vi "SubVI_EncTempl_003.vi"(0 "Encoder parameters":T1) -> (1 "Template images":picture[](array[picture]), 2 "Cluster templates":cluster{i32[], i32[][]})   [LabVIEW 2018]
panel:
  out "spike index array":i32[][](array[numeric])
  out "total spikes array":i32[](array[numeric])
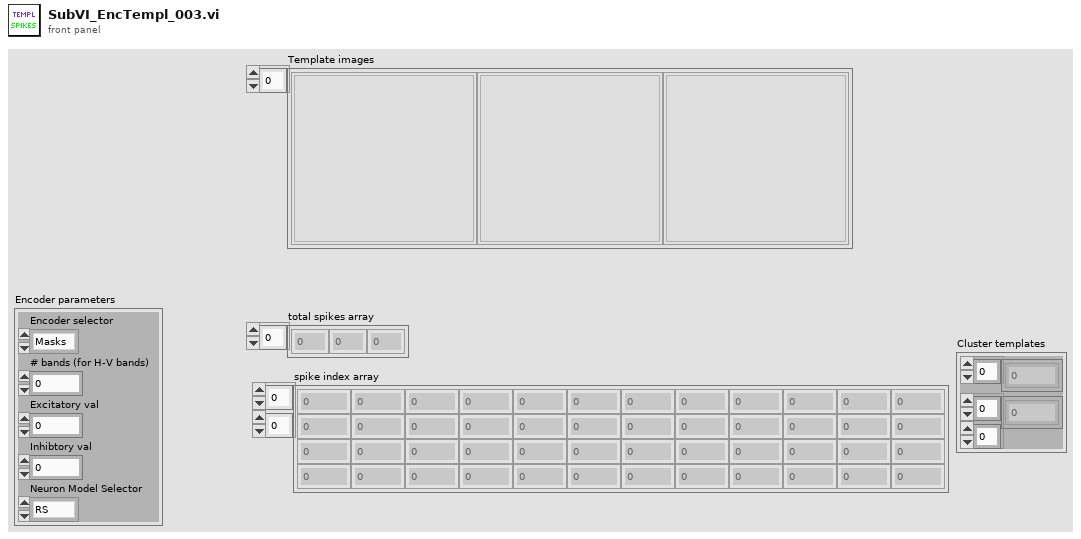
[diagram p1: front panel]
types:
  T1 = cluster{"Encoder selector":enum16{"Masks", "H-V bands", "Simple reading"}, "# bands (for H-V bands)":i32, "Excitatory val":dbl, "Inhibtory val":dbl, "Neuron Model Selector":enum16{"RS", "LTS", "RZ", "TC2", "TC1", "FS", "CH", "IB"}}
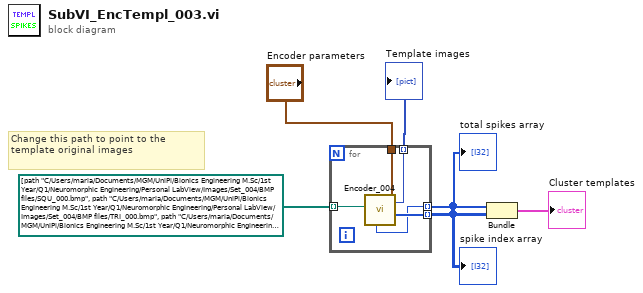
[diagram p0: block diagram]
diagram:
  # "Change this path to point to the template original images"
  n1 = for {
    tunnel: "Encoder parameters" -> [w11]
    tunnel: path[] [path "C:/Users/maria/Documents/MGM/UniPi/Bionics Engineering M.Sc/1st Year/Q1/Neuromorphic Engineering/Personal LabView/Images/Set_004/BMP files/SQU_000.bmp", path "C:/Users/maria/Documents/MGM/UniPi/Bionics Engineering M.Sc/1st Year/Q1/Neuromorphic Engineering/Personal LabView/Images/Set_004/BMP files/TRI_000.bmp", path "C:/Users/maria/Documents/MGM/UniPi/Bionics Engineering M.Sc/1st Year/Q1/Neuromorphic Engineering/Personal LabView/Images/Set_004/BMP files/CIR_000.bmp"] ("Array") -> [w10] mode=indexing
    tunnel: [w8] -> w4 mode=indexing
    tunnel: [w7] -> w3 mode=indexing
    tunnel: [w9] -> w1 mode=indexing
    n2 = call "Encoder_004.vi"("Image Path"=w10, "Encoder parameters"=w11) -> ("spike indexes"=w9:i32[], "total duration"=w7:i32, "Picture"=w8:picture)  [unwired: 4 in, 3 out]
  }
  "Template images" <- w4
  "spike index array" <- w1
  "total spikes array" <- w3
  n3 = Bundle(w3, "spike indexes"=w1) -> (→"Cluster templates":cluster{i32[], "spike indexes":i32[][]})  [unwired: 1 in]
